vi "GFITS_Fits2File.vi"(7 "write to file?":bool=TRUE, 8 "error in (no error)":errorcluster, 9 "Keywords":string[][](array[string])=[["DATE-OBS", "unknown", "' /Date (dd/mm/yy) of observation"], ["UT", "unknown", "' /UT of TCS coordinates"], ["RA", "unknown", "' /right ascension (telescope)"], ["DEC", "unknown", "' /declination (telescope)"], ["EQUINOX", "unknown", "' /epoch of RA & DEC"], ["HA", "unknown", "' /hour angle (H:M:S)"], ["ST", "unknown", "' /siderial time"], ["AIRMASS", "unknown", "' /airmass"], ["ZD", "unknown", "' /zenith distance (degrees)"], ["TELFOCUS", "unknown", "' /Telescope focus"], ["FILTNUM", "unknown", "' /Filter number"], ["FILTERS", "unknown", "' /Selected Filter name"], ["", "", ""], ["", "", ""], ["", "", ""], ["", "", ""], ["", "", ""], ["", "", ""], ["", "", ""], ["", "", ""], ["", "", ""], ["", "", ""]], 10 "append to file? (new file:F)":bool=TRUE, 11 "filename":path) -> (0 "error out":errorcluster, 2 "string out":string)   [LabVIEW 2016]
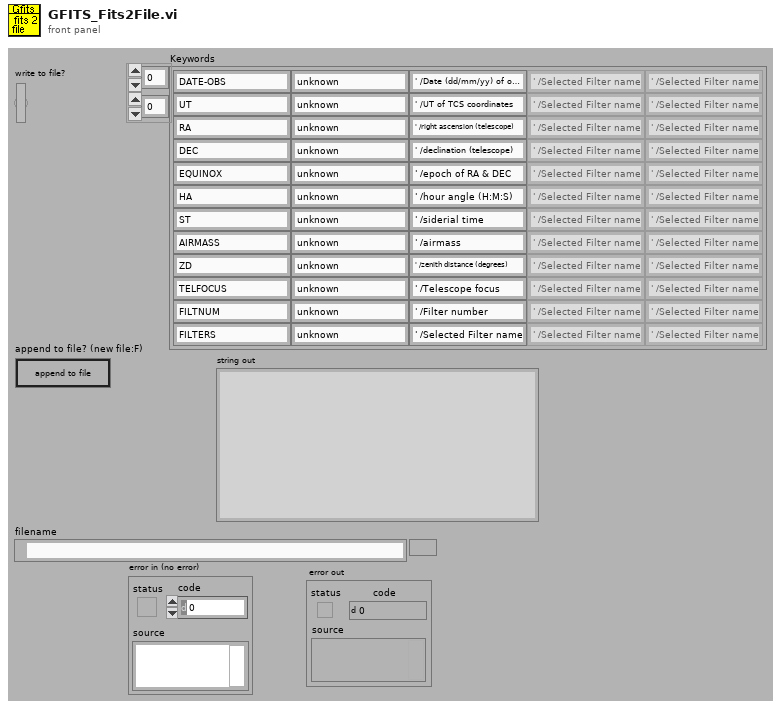
[diagram p1: front panel]
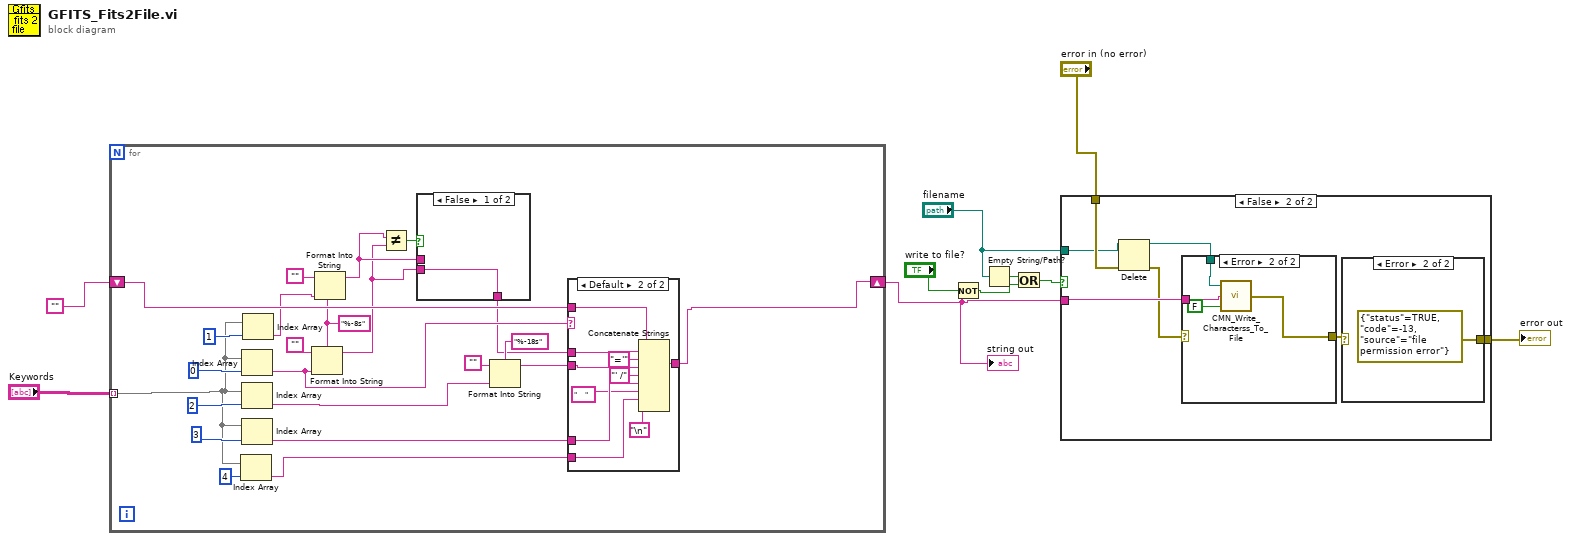
[diagram p0: block diagram]
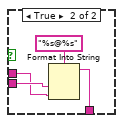
[diagram p2: hidden frame]
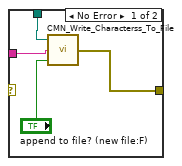
[diagram p6: hidden frame]
diagram:
  n1 = for {
    tunnel: "Keywords" -> [w13] mode=indexing
    shift-right: [w33] -> w9
    shift-left: "" -> [w22]
    w18 = "%-8s" ("Format String")
    n2 = Index Array(array=w13, index=4) -> (element=w11:string)
    n3 = Index Array(array=w13, index=0 ("Index")) -> (element=w24:string)
    n4 = Index Array(array=w13, index=2 ("Index")) -> (element=w23:string)
    n5 = Index Array(array=w13, index=3 ("Index")) -> (element=w25:string)
    n6 = Index Array(array=w13, index=1) -> (element=w20:string)
    n7 = Format Into String(format string=w18, initial string="", w24) -> (resulting string=w15:string)  [unwired: 1 in, 1 out]
    n8 = Format Into String(format string=w18, initial string="", w20) -> (resulting string=w16:string)  [unwired: 1 in, 1 out]
    n9 = Not Equal?(x=w16, y=w15) -> (x != y?=w17:bool)
    n10 = case shown="False" w17 {
      tunnel: w16 -> [_ w36]
      tunnel: w15 -> [w34 w37]
      tunnel: [w34 w35] -> w14
      frame False {
      }
      frame True {
        n11 = Format Into String(format string="%s@%s", w37, w36) -> (resulting string=w35:string)  [unwired: 2 in, 1 out]
      }
    }
    n12 = Format Into String(format string="%-18s" ("Format String"), initial string="", w23) -> (resulting string=w26:string)  [unwired: 1 in, 1 out]
    n13 = case shown="Default" w24 {
      tunnel: w22 -> [w39 w49]
      tunnel: [w39 w48] -> w33
      tunnel: w14 -> [_ w47]
      tunnel: w26 -> [_ w45]
      tunnel: w25 -> [_ w43]
      tunnel: w11 -> [_ w41]
      frame "", " " {
      }
      frame Default {
        n14 = Concatenate Strings(w49, w47, "='" ("Substring"), w45, "' /" ("Substring"), w43, "    " ("string"), w41, "\n") -> (w48:string)
      }
    }
  }
  "string out" <- w9
  n15 = Not(x="write to file?") -> (.not. x?=w2:bool)
  n16 = Empty String/Path?(string/path="filename") -> (empty?=w4:bool)
  n17 = Or(x=w4, y=w2) -> (x .or. y?=w5:bool)
  n18 = case shown="False" w5 {
    tunnel: w9 -> [_ w57]
    tunnel: "filename" -> [_ w55]
    tunnel: [w50 w51] -> w1
    tunnel: "error in (no error)" -> [w50 w56]
    frame True {
    }
    frame False {
      n19 = Delete(path (use dialog)=w55, error in=w56) -> (deleted path=w54:path, error out=w53:errorcluster)  [unwired: 4 out]
      n20 = case shown="Error" w53 {
        tunnel: w57 -> [w63 w67]
        tunnel: w54 -> [w61 w66]
        tunnel: [w60 w65] -> w52
        frame No Error {
          n21 = call "CMN_Write_Characterss_To_File.vi"("append to file? (new file:F)"="append to file? (new file:F)", "character string"=w63, "file path (dialog if empty)"=w61) -> ("error out"=w60:errorcluster)  [unwired: 2 out]
        }
        frame Error {
          n22 = call "CMN_Write_Characterss_To_File.vi"("append to file? (new file:F)"=FALSE, "character string"=w67, "file path (dialog if empty)"=w66) -> ("error out"=w65:errorcluster)  [unwired: 2 out]
        }
      }
      n23 = case shown="Error" w52 {
        selector: w52 -> [w58 _]
        tunnel: [w58 errorcluster {"status"=TRUE, "code"=-13, "source"="file permission error"} ("error IO")] -> w51
        frame No Error {
        }
        frame Error {
        }
      }
    }
  }
  "error out" <- w1
